vi "ClearDependencies.vi"(8 "error in (no error)":errorcluster, 11 "SMO in":refnum<class "SMO.lvclass">) -> (0 "error out":errorcluster, 3 "SMO out":refnum<class "SMO.lvclass">)   [LabVIEW 2013, in "SMO.lvclass"]
uses:
  SMO.lvclass
  Support/Attribute.Dependencies/Attribute.Dependencies.lvclass
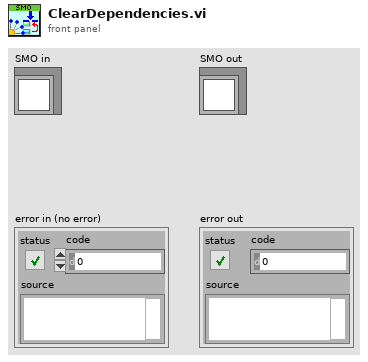
[diagram p1: front panel]
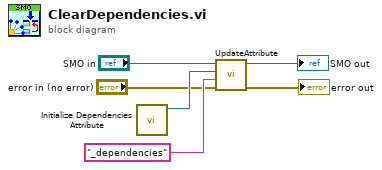
[diagram p0: block diagram]
diagram:
  n1 = call "Initialize Dependencies Attribute.vi"() -> ("Attribute.Dependencies"=w5:refnum<class "Attribute.Dependencies.lvclass">)  [unwired: 11 in]
  n2 = call "UpdateAttribute.vi"("error in (no error)"="error in (no error)", "Attribute Name"="_dependencies" ("name"), "Attribute"=w5, "SMO in"="SMO in") -> ("error out"=→"error out":errorcluster, "SMO out"=→"SMO out":refnum<class "SMO.lvclass">)  [unwired: 5 in, 1 out]
